vi "Calculate Velocity Setpoints.vi"(0 "Negated":bool, 1 "Front is Back":bool, 3 "Reversed":bool, 4 "Iterations":i32, 5 "Time":u32, 6 "Velocity Data":dbl[](array[numeric]), 7 "Angular Data (Relative)":dbl[](array[numeric]), 8 "f":dbl=0.17 format="%#_13g", 9 "Align?":bool, 10 "PID gains L/S 2":T1={"proportional gain (Kc)"=0.08, "integral time (Ti, min)"=0.0, "derivative time (Td, min)"=0.001} {"derivative time (Td, min)" format="%.3e"; "integral time (Ti, min)" format="%.3e"; "proportional gain (Kc)" format="%#.6e"}, 11 "Enum":enum16{"Vantage", "Mule", "Linda/Sophie"}(ring), 12 "Angle To Get":dbl(slide) scale=0.0..360.0, 13 "IMU Input":dbl) -> (14 "Left Setpoint":dbl, 15 "Wait Time (ms)":dbl, 18 "Finished?":bool, 19 "Right Setpoint":dbl)   [LabVIEW 2018]
doc: "Converting velocity and angle setpoints to left and right setpoints on the robot"
uses:
  <vilib>/addons/control/pid/pid.llb/PID (DBL).vi
  <vilib>/addons/control/pid/NI_PID_pid.lvlib
panel:
  out "Angles PID L/S":cluster{"Numeric":dbl, "IMU Input":dbl}(graph)
  out "Angles PID M":cluster{"Numeric":dbl, "IMU Input":dbl}(graph)
  out "Timing Feedback":u32(graph)
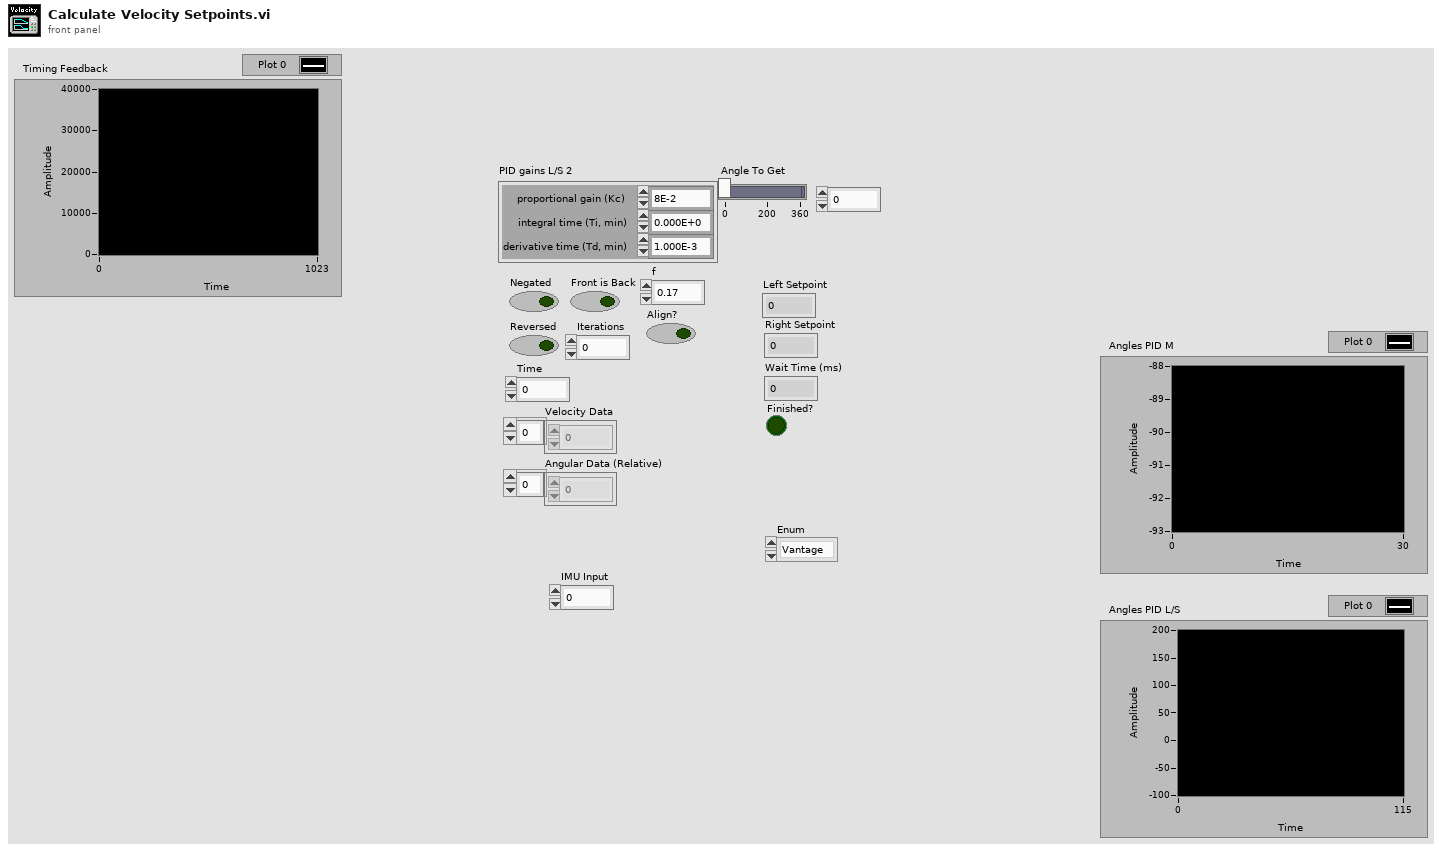
[diagram p1: front panel]
types:
  T1 = cluster{"proportional gain (Kc)":dbl, "integral time (Ti, min)":dbl, "derivative time (Td, min)":dbl}
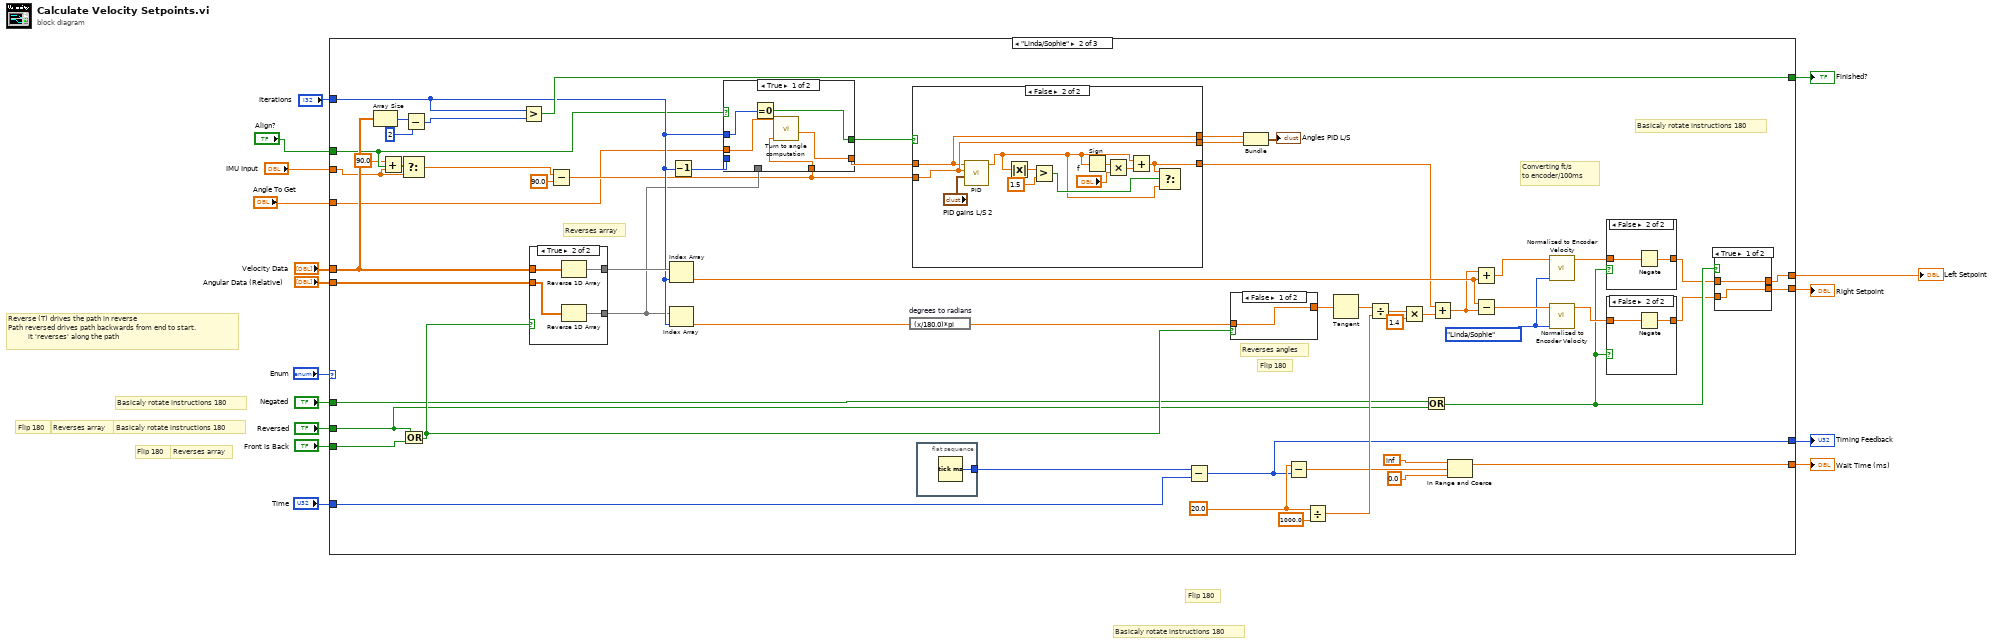
[diagram p0: block diagram]
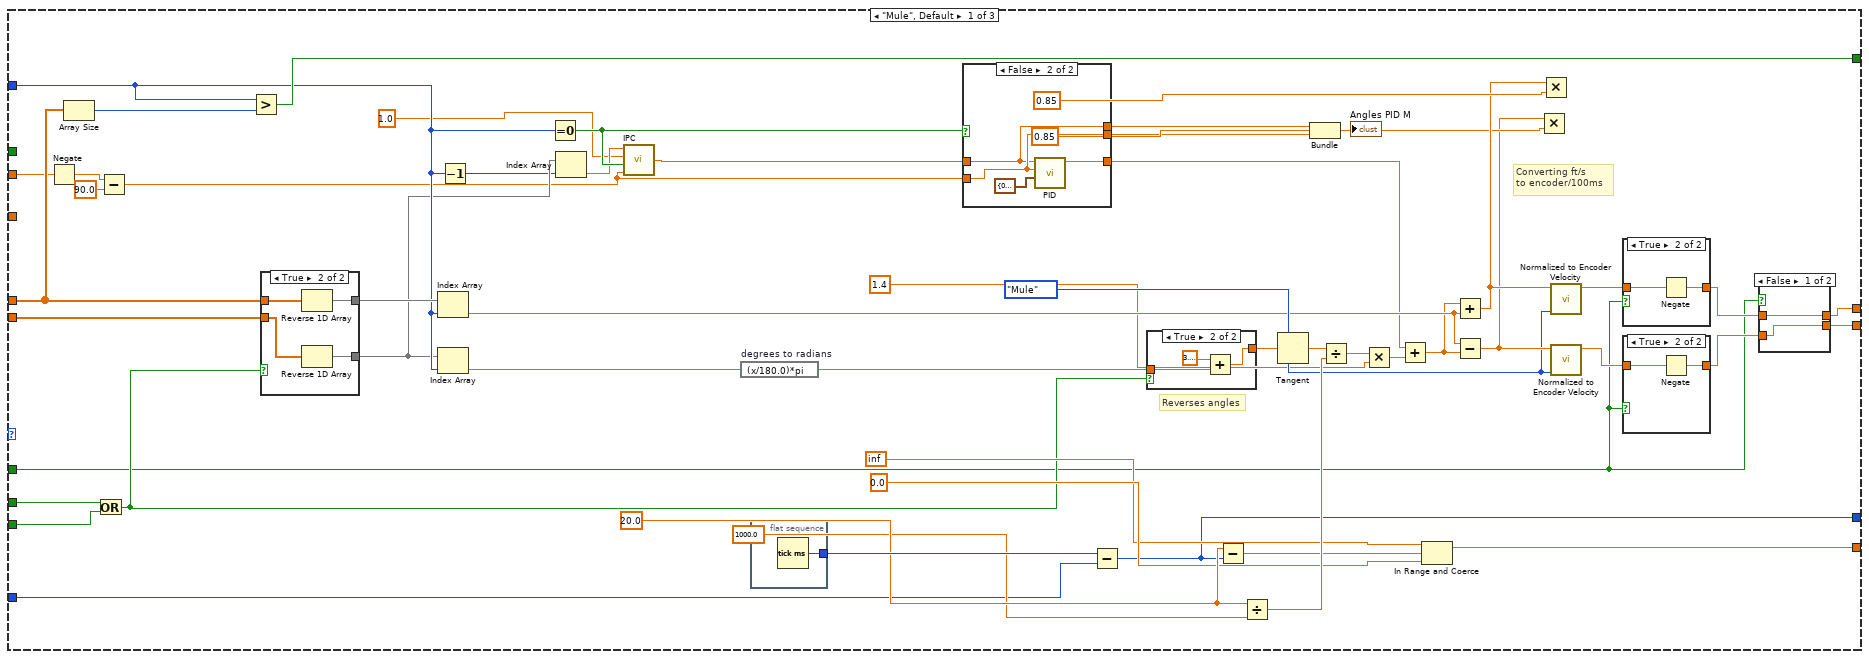
[diagram p2: hidden frame]
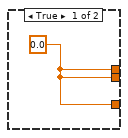
[diagram p3: hidden frame]
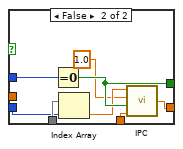
[diagram p9: hidden frame]
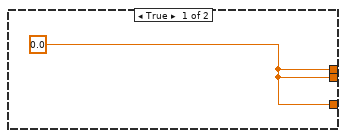
[diagram p10: hidden frame]
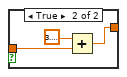
[diagram p13: hidden frame]
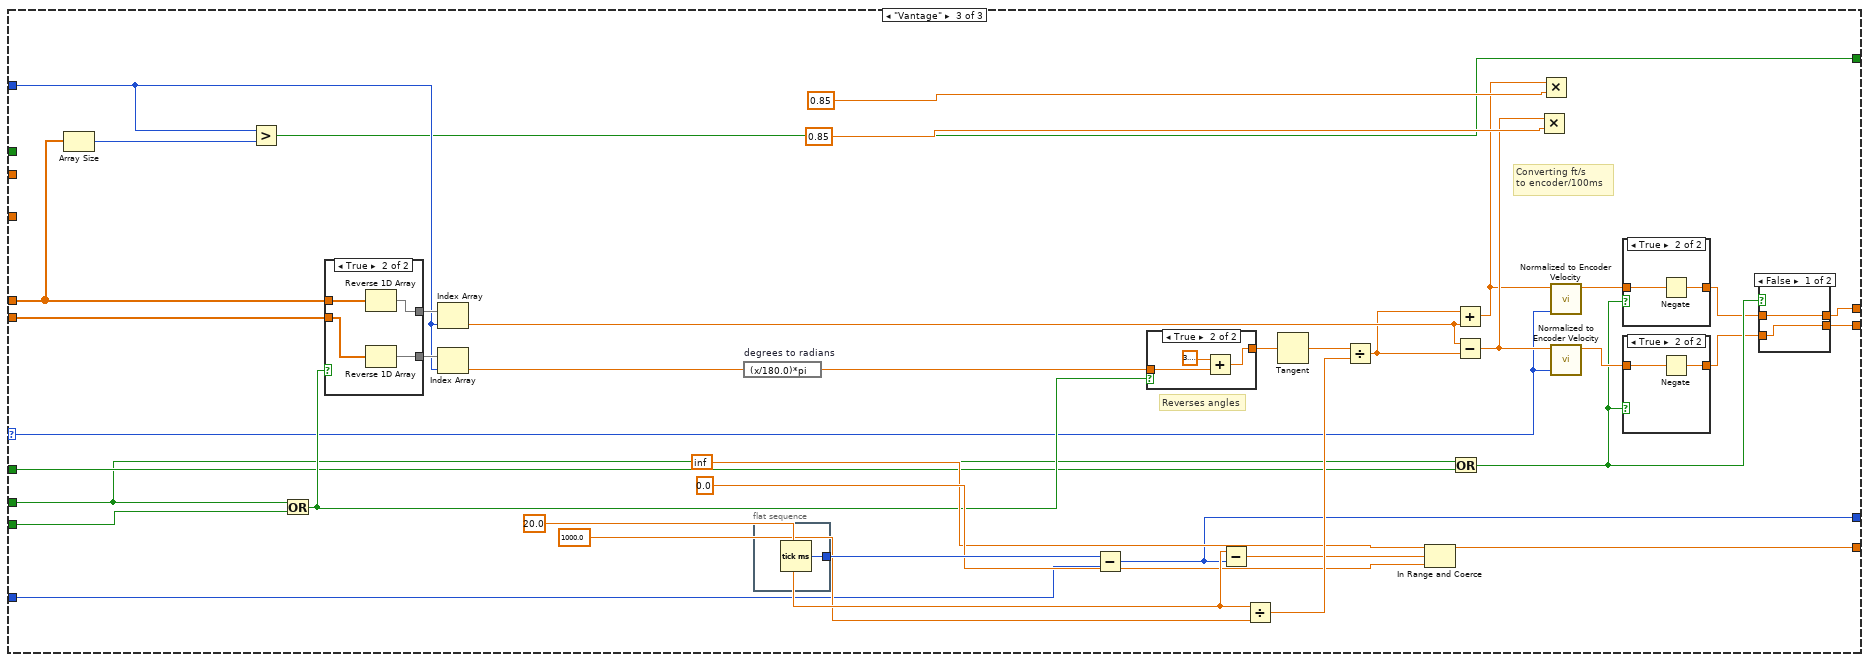
[diagram p16: hidden frame]
diagram:
  # "Reverse (T) drives the path in reverse\nPath reversed drives path backwards from end to start. \n          it 'reverses' along the path"
  # "Basicaly rotate instructions 180"
  # "Basicaly rotate instructions 180"
  # "Flip 180"
  # "Flip 180"
  # "Reverses array"
  # "Reverses array"
  # "Flip 180"
  # "Basicaly rotate instructions 180"
  n1 = case shown="\"Linda/Sophie\"" "Enum" {
    selector: "Enum" -> [_ _ w200]
    tunnel: "Negated" -> [w17 w137 w216]
    tunnel: "Reversed" -> [w54 w136 w215]
    tunnel: "Front is Back" -> [w53 w135 w214]
    tunnel: "Iterations" -> [w26 w114 w213]
    tunnel: "Time" -> [w52 w134 w212]
    tunnel: "Angular Data (Relative)" -> [w51 w133 w211]
    tunnel: "Velocity Data" -> [w50 w132 w210]
    tunnel: [w45 w129 w206] -> w8
    tunnel: [w44 w128 w205] -> w3
    tunnel: [w43 w127 w204] -> w7
    tunnel: [w42 w126 w203] -> w6
    tunnel: [w41 w125 w202] -> w5
    tunnel: "IMU Input" -> [w29 w99 _]
    tunnel: "Align?" -> [_ w102 _]
    tunnel: "Angle To Get" -> [_ w103 _]
    frame "Mule", Default {
      w40 = enum16{"Vantage", "Mule"}."Mule" ("Enum")
      w68 = 20.0 ("x")
      # "Converting ft/s\nto encoder/100ms"
      # "Reverses angles"
      n2 = Negate(x=w29) -> (-x=w28:dbl)
      n3 = Array Size(array=w50) -> (size(s)=w58:i32)
      n4 = Or(x=w54, y=w53) -> (x .or. y?=w57:bool)
      n5 = Subtract(x=w28, y=90.0) -> (x-y=w20:dbl)
      n6 = Greater?(x=w26, y=w58) -> (0:w41:bool)
      n7 = case shown="True" w57 {
        tunnel: [w80 w85] -> w25
        tunnel: [w81 w84] -> w59
        tunnel: w51 -> [w80 w82]
        tunnel: w50 -> [w81 w83]
        frame False {
        }
        frame True {
          n8 = Reverse 1D Array(array=w83) -> (reversed array=w84:dbl[])
          n9 = Reverse 1D Array(array=w82) -> (reversed array=w85:dbl[])
        }
      }
      n10 = Index Array(array=w59, index=w26) -> (element=w39:dbl)
      n11 = Index Array(array=w25, index=w26) -> (element=w37:dbl)
      n12 = Decrement(x=w26) -> (x-1=w24:i32)
      n13 = Equal To 0?(x=w26) -> (x = 0?=w23:bool)
      n14 = Index Array(array=w25, index=w24) -> (element=w22:dbl)
      n15 = call "IPC.vi"("Initilization"=w20, "Reset"=w23, "Multiplier"=1.0, "Value"=w22) -> ("IPCed"=w21:dbl)  [unwired: 2 in]
      n16 = expression code="(x/180.0)*pi" "degrees to radians"(w37) -> (w36:dbl)
      n17 = flat-sequence {
        tunnel: [w96] -> w70
        frame #0 {
          n18 = Tick Count (ms)() -> (millisecond timer value=w96:u32)
        }
      }
      n19 = case shown="False" w23 {
        tunnel: w20 -> [_ w73]
        tunnel: [w71 w74] -> w18
        tunnel: [w71 w72] -> w31
        tunnel: [w71 w73] -> w30
        tunnel: w21 -> [_ w72]
        frame True {
          w71 = 0.0 ("output")
        }
        frame False {
          n20 = call-poly <vilib>:"PID.vi"("PID gains"=T1 {"proportional gain (Kc)"=0.2, "integral time (Ti, min)"=0.4, "derivative time (Td, min)"=0.0006} ("PID gains M"), "process variable"=w73, "setpoint"=w72) -> ("output"=w74:dbl)  [unwired: 7 in, 1 out]
        }
      }
      n21 = Subtract(x=w70, y=w52) -> (x-y=w42:u32)
      n22 = case shown="True" w57 {
        tunnel: w36 -> [w86 w89]
        tunnel: [w86 w88] -> w60
        frame False {
        }
        frame True {
          n23 = Add(x=3.141592653589793, y=w89) -> (x+y=w88:dbl)
        }
      }
      n24 = Subtract(x=w68, y=w42) -> (x-y=w64:dbl)
      n25 = Divide(x=w68, y=1000.0) -> (x/y=w66:dbl)
      n26 = Tangent(1:w60) -> (0:w69:dbl)
      n27 = Bundle("IPCed"=w31, "output"=w30) -> (→"Angles PID M":cluster{"IPCed":dbl, "output":dbl})  [unwired: 1 in]
      n28 = Divide(x=w69, y=w66) -> (x/y=w38:dbl)
      n29 = Multiply(x=w38, y=1.4) -> (x*y=w34:dbl)
      n30 = Add(x=w18, y=w34) -> (x+y=w33:dbl)
      n31 = In Range and Coerce(upper limit=inf, x=w64, lower limit=0.0) -> (coerced(x)=w43:dbl)  [unwired: 1 out]
      n32 = Add(x=w33, y=w39) -> (x+y=w48:dbl)
      n33 = Subtract(x=w39, y=w33) -> (x-y=w46:dbl)
      n34 = Multiply(x=w46, y=0.85) -> ()  [unwired: 1 out]
      n35 = Multiply(x=w48, y=0.85) -> ()  [unwired: 1 out]
      n36 = call "Normalized to Encoder Velocity.vi"("Enum"=w40, "ft/s"=w48) -> ("Output"=w62:dbl)  [unwired: 9 in]
      n37 = call "Normalized to Encoder Velocity.vi"("Enum"=w40, "ft/s"=w46) -> ("Output"=w61:dbl)  [unwired: 9 in]
      n38 = case shown="True" w17 {
        tunnel: w62 -> [w93 w95]
        tunnel: [w93 w94] -> w56
        frame False {
        }
        frame True {
          n39 = Negate(x=w95) -> (-x=w94:dbl)
        }
      }
      n40 = case shown="True" w17 {
        tunnel: [w90 w92] -> w55
        tunnel: w61 -> [w90 w91]
        frame False {
        }
        frame True {
          n41 = Negate(x=w91) -> (-x=w92:dbl)
        }
      }
      n42 = case shown="False" w17 {
        tunnel: w55 -> [w77 w78]
        tunnel: w56 -> [w76 w79]
        tunnel: [w77 w79] -> w45
        tunnel: [w76 w78] -> w44
        frame False {
        }
        frame True {
        }
      }
    }
    frame "Linda/Sophie" {
      w108 = enum16{"Vantage", "Mule", "Linda/Sophie"}."Linda/Sophie" ("Enum")
      w151 = 20.0 ("x")
      # "Basicaly rotate instructions 180"
      # "Flip 180"
      # "Reverses array"
      # "Converting ft/s\nto encoder/100ms"
      # "Reverses angles"
      n43 = Array Size(array=w132) -> (size(s)=w106:i32)
      n44 = Add(x=90.0, y=w99) -> (x+y=w100:dbl)
      n45 = Select(t=w100, s=w102, f=w99) -> (s? t:f=w97:dbl)
      n46 = Or(x=w136, y=w135) -> (x .or. y?=w141:bool)
      n47 = Subtract(x=w106, y=2) -> (x-y=w105:i32)
      n48 = Greater?(x=w114, y=w105) -> (0:w125:bool)
      n49 = case shown="True" w141 {
        tunnel: [w183 w188] -> w113
        tunnel: [w184 w187] -> w142
        tunnel: w133 -> [w183 w185]
        tunnel: w132 -> [w184 w186]
        frame False {
        }
        frame True {
          n50 = Reverse 1D Array(array=w186) -> (reversed array=w187:dbl[])
          n51 = Reverse 1D Array(array=w185) -> (reversed array=w188:dbl[])
        }
      }
      n52 = Subtract(x=w97, y=90.0) -> (x-y=w109:dbl)
      n53 = Index Array(array=w142, index=w114) -> (element=w124:dbl)
      n54 = Index Array(array=w113, index=w114) -> (element=w122:dbl)
      n55 = Decrement(x=w114) -> (x-1=w112:i32)
      n56 = case shown="True" w102 {
        tunnel: w114 -> [w155 w166]
        tunnel: w113 -> [_ w165]
        tunnel: w112 -> [_ w164]
        tunnel: [w154 w163] -> w111
        tunnel: [w156 w161] -> w110
        tunnel: w109 -> [w158 w160]
        tunnel: w103 -> [w157 _]
        frame True {
          n57 = Equal To 0?(x=w155) -> (x = 0?=w154:bool)
          n58 = call "Turn to angle computation.vi"("Current Angle"=w158, "Angle To Get"=w157) -> ("Current Angle 2"=w156:dbl)  [unwired: 9 in]
        }
        frame False {
          n59 = Equal To 0?(x=w166) -> (x = 0?=w163:bool)
          n60 = Index Array(array=w165, index=w164) -> (element=w162:dbl)
          n61 = call "IPC.vi"("Initilization"=w160, "Reset"=w163, "Multiplier"=1.0, "Value"=w162) -> ("IPCed"=w161:dbl)  [unwired: 2 in]
        }
      }
      n62 = expression code="(x/180.0)*pi" "degrees to radians"(w122) -> (w121:dbl)
      n63 = case shown="False" w111 {
        tunnel: w109 -> [_ w178]
        tunnel: [w167 w171] -> w107
        tunnel: [w167 w177] -> w116
        tunnel: [w167 w178] -> w115
        tunnel: w110 -> [_ w177]
        frame True {
          w167 = 0.0 ("output")
        }
        frame False {
          n64 = call-poly <vilib>:"PID.vi"("PID gains"="PID gains L/S 2", "process variable"=w178, "setpoint"=w177) -> ("output"=w169:dbl)  [unwired: 7 in, 1 out]
          n65 = Absolute Value(x=w169) -> (abs(x)=w173:dbl)
          n66 = Greater?(x=w173, y=1.5) -> (0:w170:bool)
          n67 = Sign(1:w169) -> (0:w176:dbl)
          n68 = Multiply(x=w176, y="f") -> (x*y=w175:dbl)
          n69 = Add(x=w169, y=w175) -> (x+y=w171:dbl)
          n70 = Select(t=w171, s=w170, f=w169) -> ()  [unwired: 1 out]
        }
      }
      n71 = flat-sequence {
        tunnel: [w199] -> w153
        frame #0 {
          n72 = Tick Count (ms)() -> (millisecond timer value=w199:u32)
        }
      }
      n73 = Subtract(x=w153, y=w134) -> (x-y=w126:u32)
      n74 = case shown="False" w141 {
        tunnel: w121 -> [w189 w192]
        tunnel: [w189 w191] -> w143
        frame False {
        }
        frame True {
          n75 = Add(x=3.141592653589793, y=w192) -> (x+y=w191:dbl)
        }
      }
      n76 = Bundle("IPCed"=w116, "output"=w115) -> (→"Angles PID L/S":cluster{"IPCed":dbl, "output":dbl})  [unwired: 1 in]
      n77 = Subtract(x=w151, y=w126) -> (x-y=w147:dbl)
      n78 = Divide(x=w151, y=1000.0) -> (x/y=w149:dbl)
      n79 = Tangent(1:w143) -> (0:w152:dbl)
      n80 = Divide(x=w152, y=w149) -> (x/y=w123:dbl)
      n81 = Multiply(x=w123, y=1.4) -> (x*y=w119:dbl)
      n82 = Or(x=w137, y=w136) -> (x .or. y?=w140:bool)
      n83 = Add(x=w107, y=w119) -> (x+y=w118:dbl)
      n84 = In Range and Coerce(upper limit=inf, x=w147, lower limit=0.0) -> (coerced(x)=w127:dbl)  [unwired: 1 out]
      n85 = Add(x=w118, y=w124) -> (x+y=w131:dbl)
      n86 = Subtract(x=w124, y=w118) -> (x-y=w130:dbl)
      n87 = call "Normalized to Encoder Velocity.vi"("Enum"=w108, "ft/s"=w131) -> ("Output"=w145:dbl)  [unwired: 9 in]
      n88 = call "Normalized to Encoder Velocity.vi"("Enum"=w108, "ft/s"=w130) -> ("Output"=w144:dbl)  [unwired: 9 in]
      n89 = case shown="False" w140 {
        tunnel: w145 -> [w196 w198]
        tunnel: [w196 w197] -> w139
        frame True {
        }
        frame False {
          n90 = Negate(x=w198) -> (-x=w197:dbl)
        }
      }
      n91 = case shown="False" w140 {
        tunnel: [w193 w195] -> w138
        tunnel: w144 -> [w193 w194]
        frame True {
        }
        frame False {
          n92 = Negate(x=w194) -> (-x=w195:dbl)
        }
      }
      n93 = case shown="True" w140 {
        tunnel: w138 -> [w180 w181]
        tunnel: w139 -> [w179 w182]
        tunnel: [w180 w182] -> w129
        tunnel: [w179 w181] -> w128
        frame True {
        }
        frame False {
        }
      }
    }
    frame "Vantage" {
      w234 = 20.0 ("x")
      # "Converting ft/s\nto encoder/100ms"
      # "Reverses angles"
      n94 = Array Size(array=w210) -> (size(s)=w221:i32)
      n95 = Greater?(x=w213, y=w221) -> (0:w202:bool)
      n96 = Or(x=w215, y=w214) -> (x .or. y?=w220:bool)
      n97 = case shown="True" w220 {
        tunnel: [w243 w248] -> w224
        tunnel: [w244 w247] -> w223
        tunnel: w211 -> [w243 w245]
        tunnel: w210 -> [w244 w246]
        frame False {
        }
        frame True {
          n98 = Reverse 1D Array(array=w246) -> (reversed array=w247:dbl[])
          n99 = Reverse 1D Array(array=w245) -> (reversed array=w248:dbl[])
        }
      }
      n100 = Index Array(array=w223, index=w213) -> (element=w237:dbl)
      n101 = Index Array(array=w224, index=w213) -> (element=w222:dbl)
      n102 = expression code="(x/180.0)*pi" "degrees to radians"(w222) -> (w226:dbl)
      n103 = flat-sequence {
        tunnel: [w259] -> w238
        frame #0 {
          n104 = Tick Count (ms)() -> (millisecond timer value=w259:u32)
        }
      }
      n105 = Subtract(x=w238, y=w212) -> (x-y=w203:u32)
      n106 = case shown="True" w220 {
        tunnel: w226 -> [w249 w252]
        tunnel: [w249 w251] -> w225
        frame False {
        }
        frame True {
          n107 = Add(x=3.141592653589793, y=w252) -> (x+y=w251:dbl)
        }
      }
      n108 = Subtract(x=w234, y=w203) -> (x-y=w230:dbl)
      n109 = Divide(x=w234, y=1000.0) -> (x/y=w232:dbl)
      n110 = Tangent(1:w225) -> (0:w236:dbl)
      n111 = Divide(x=w236, y=w232) -> (x/y=w235:dbl)
      n112 = In Range and Coerce(upper limit=inf, x=w230, lower limit=0.0) -> (coerced(x)=w204:dbl)  [unwired: 1 out]
      n113 = Or(x=w215, y=w216) -> (x .or. y?=w219:bool)
      n114 = Add(x=w235, y=w237) -> (x+y=w201:dbl)
      n115 = Subtract(x=w237, y=w235) -> (x-y=w207:dbl)
      n116 = Multiply(x=w207, y=0.85) -> ()  [unwired: 1 out]
      n117 = Multiply(x=w201, y=0.85) -> ()  [unwired: 1 out]
      n118 = call "Normalized to Encoder Velocity.vi"("Enum"=w200, "ft/s"=w201) -> ("Output"=w228:dbl)  [unwired: 9 in]
      n119 = call "Normalized to Encoder Velocity.vi"("Enum"=w200, "ft/s"=w207) -> ("Output"=w227:dbl)  [unwired: 9 in]
      n120 = case shown="True" w219 {
        tunnel: w228 -> [w256 w258]
        tunnel: [w256 w257] -> w218
        frame False {
        }
        frame True {
          n121 = Negate(x=w258) -> (-x=w257:dbl)
        }
      }
      n122 = case shown="True" w219 {
        tunnel: [w253 w255] -> w217
        tunnel: w227 -> [w253 w254]
        frame False {
        }
        frame True {
          n123 = Negate(x=w254) -> (-x=w255:dbl)
        }
      }
      n124 = case shown="False" w219 {
        tunnel: w217 -> [w240 w241]
        tunnel: w218 -> [w239 w242]
        tunnel: [w240 w242] -> w206
        tunnel: [w239 w241] -> w205
        frame False {
        }
        frame True {
        }
      }
    }
  }
  "Left Setpoint" <- w3
  "Right Setpoint" <- w8
  "Wait Time (ms)" <- w7
  "Timing Feedback" <- w6
  "Finished?" <- w5
